vi "Draw.vi"(1 "数组":u8[][](array[numeric]), 2 "point":cluster{"x":i16, "y":i16}, 3 "背景图片":picture) -> (0 "输出":picture)   [LabVIEW 2016]
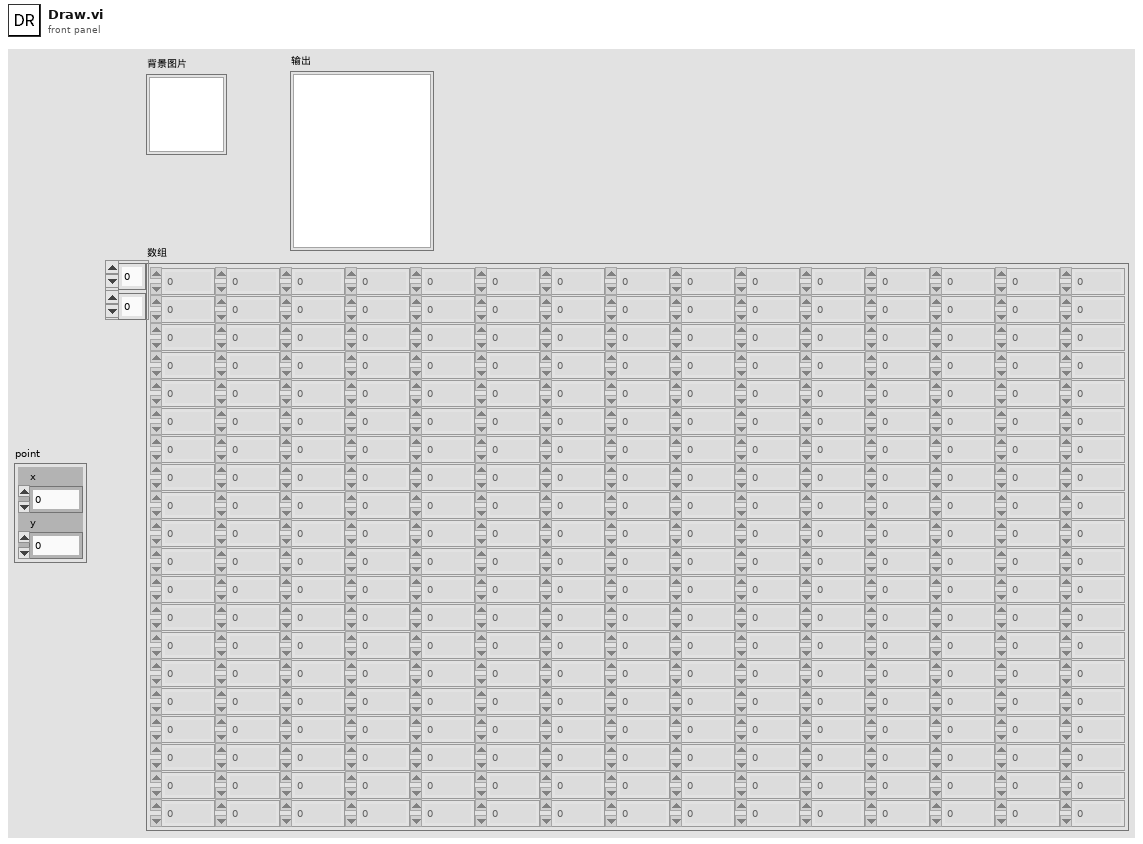
[diagram p1: front panel]
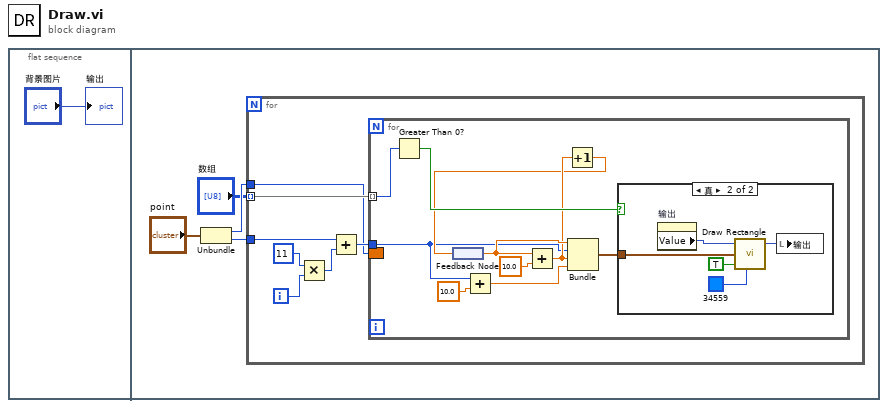
[diagram p0: block diagram]
diagram:
  n1 = flat-sequence {
    frame #0 {
      "输出" <- "背景图片"
    }
    frame #1 {
      n2 = Unbundle("point") -> ("x"=w4:i16, "y"=w5:i16)
      n3 = for {
        tunnel: "数组" -> [w12] mode=indexing
        tunnel: w4 -> [w6]
        tunnel: w5 -> [w7]
        i -> [w11]
        n4 = Multiply(x=11, y=w11) -> (x*y=w8:i32)
        n5 = Add(x=w7, y=w8) -> (x+y=w9:i32)
        n6 = for {
          tunnel: w12 -> [w22] mode=indexing
          tunnel: w9 -> [w13]
          border: w6 -> [_]
          n7 = Greater Than 0?(x=w22) -> (x > 0?=w21:bool)
          n8 = feedback #1() -> (w17:dbl)
          n9 = Add(x=w13, y=10.0) -> (x+y=w16:dbl)
          n10 = Add(x=w17, y=10.0) -> (x+y=w15:dbl)
          n11 = Increment(x=w15) -> (x+1=w14:dbl)
          n12 = feedback-in #1(w14) -> ()
          n13 = Bundle("x"=w17, w13, w15, w16) -> (w20:cluster{"x":dbl, i32, dbl, dbl})  [unwired: 1 in]
          n14 = case shown="真" w21 {
            tunnel: w20 -> [_ w26]
            frame False {
            }
            frame True {
              n15 = property on="输出" class="Pict"() -> ("Value"=w25:picture)  [unwired: 2 in, 2 out]
              n16 = call <vilib>:"Draw Rectangle.vi"("picture"=w25, "rect"=w26, "fill?(F)"=TRUE, "color(black)"=u32 34559) -> ("new picture"=w24:picture)  [unwired: 5 in]
              n17 = local write "输出"(w24) -> ()
            }
          }
        }
      }
    }
  }
